vi "BRig_RT__Case_Exp__State_Selection.vi"(0 "input_state":T1, 2 "input_dataCurrent":u16[](array[numeric]), 3 "input_dataTrial":u16[][](array[numeric]), 4 "input_dataExp":u16[](array[numeric]), 5 "input_arrTrig":bool[](array[boolean]), 6 "input_FPGA_SelectWrong":bool, 8 "input_FPGA_SelectReward":bool, 10 "input_LickR":bool, 12 "input_LickL":bool) -> (7 "output_LC_Laser_l2":bool, 9 "output_LC_Event_l2":bool, 11 "output_LC_Laser_l1":bool, 13 "output_LC_Event_l1":bool, 14 "output_state":T1, 16 "output_dataCurrent":u16[](array[numeric]), 17 "output_dataTrial":u16[][](array[numeric]), 18 "output_anySelect_L":bool, 19 "output_anySelect_R":bool)   [LabVIEW 2014]
uses:
  myRIO_BRig_RT__Case_Exp_stateList.ctl
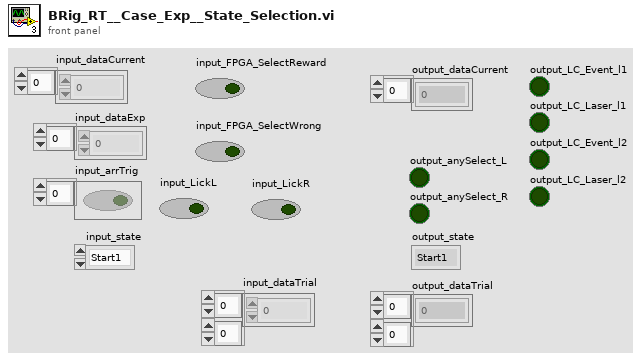
[diagram p1: front panel]
types:
  T1 = typedef "myRIO_BRig_RT__Case_Exp_stateList.ctl" = enum16{"Start1", "Start2", "Start3", "saveSettings1", "saveSettings2", "saveSettings3", "saveSettings4", "saveSettings_LC_ENL_l1", "saveSettings_LC_ENL_l2", "saveSettings_LC_Cue_l1", "saveSettings_LC_Cue_l2", "saveSettings6_LC_l1_Other", "SaveSettings6_LC_l2_Other", "setSettings_Audio", "setSettings_Laser", "initBlock_pre", "initBlock", "initBlock2", "initBlock_post", "initTrial_pre", "initTrial", "initTrial2", "initTrial3", "initTrial4", "initTrial_LC_ENL1", "initTrial_LC_Cue1", "initTrial_LC_Cue1_2", "initTrial_LC_Sel", "initTrial_post", "ENL1_pre", "ENL1", "ENL1_post", "ENL1Penalty_pre", "ENL1Penalty", "ENL2_pre", "ENL2", "ENL2Penalty_pre", "ENL2Penalty", "Cue1_pre", "Cue1", "Cue1_post", "Cue1Penalty_pre", "Cue1Penalty", "Cue2_pre", "Cue2", "Cue2Penalty_pre", "Cue2Penalty", "Selection_pre", "Selection", "Select_post", "SelectReward_pre", "SelectReward", "SelectRewardPost_pre", "SelectRewardPost", "SelectWrong_pre", "SelectWrong", "SelectWrong_post", "SelectTimeout_pre", "SelectTimeout", "SelectTimeout_post", "endTrial_pre", "endTrial1", "endTrial2", "endTrial3", "endTrial_post", "endBlock_pre", "endBlock", "endBlock_post", "endExp", "commConnect", "commUpload_pre", "commUpload_dataBlock", "commUpload_dataCurrent", "commUpload_dataExp", "commUpload_dataLC", "commUpload_dataTrial", "commUpload_post", "saveData_pre", "saveData_dataBlock", "saveData_dataCurrent", "saveData_dataExp", "saveData_dataLC", "saveData_dataTrial", "saveData_post", "empty_endBlock1", "empty_endBlock2", "empty_endTrial1", "empty_endTrial2", "empty_endTrial3", "empty_endTrial4", "empty_endTrial5", "dummyState", "dummyState_endBlock", "FreeReward_pre", "FreeReward", "FreeRewardPost_pre", "FreeRewardPost"}
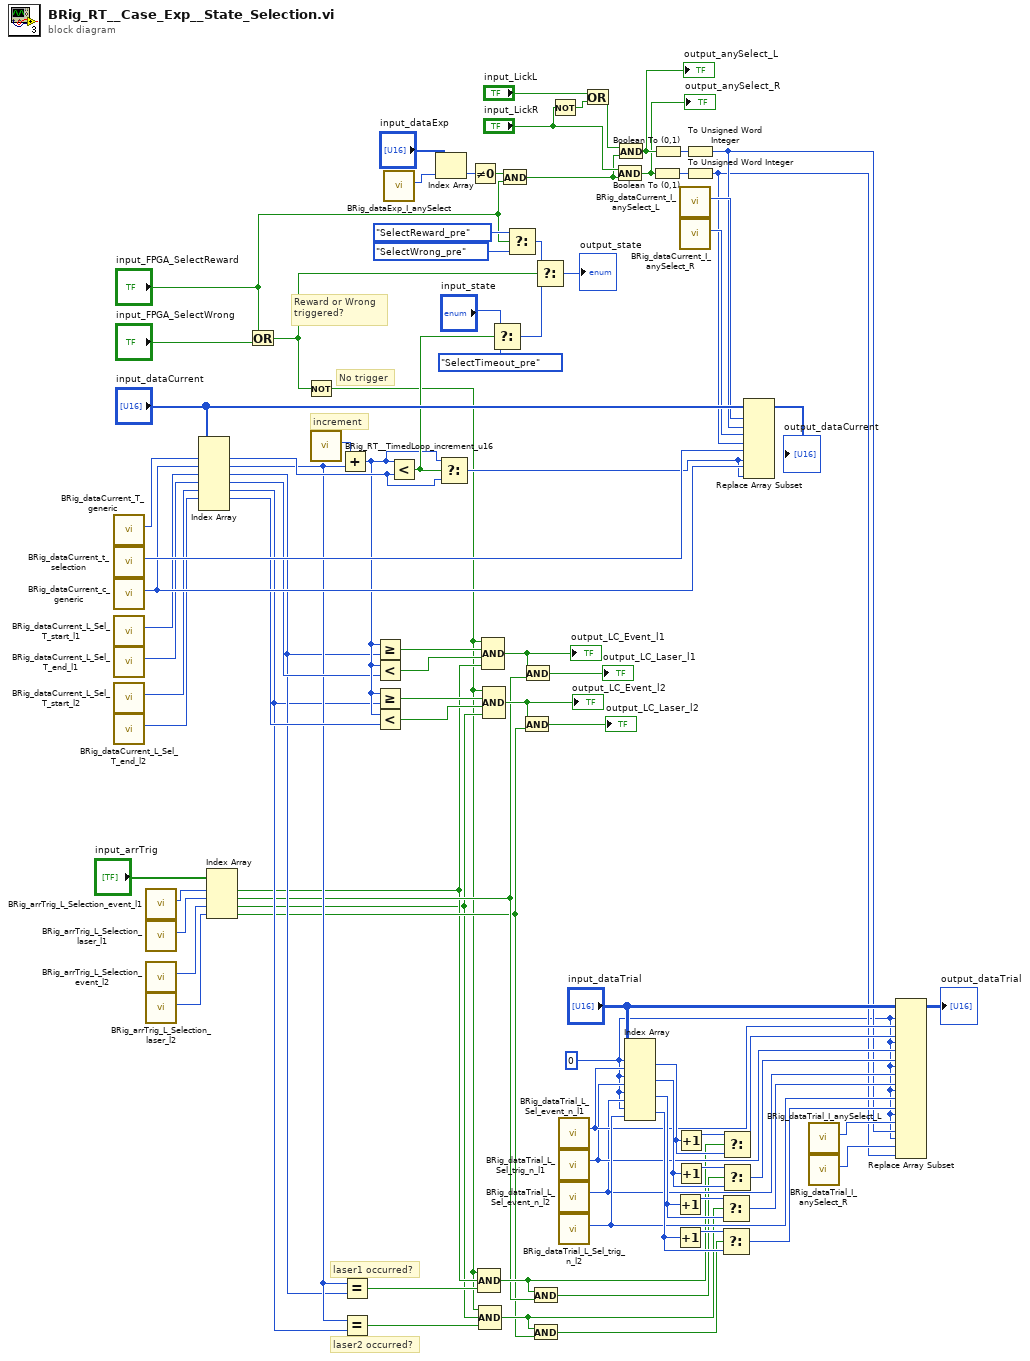
[diagram p0: block diagram]
diagram:
  w1 = 0
  # "No trigger"
  # "Reward or Wrong\ntriggered?"
  # "laser2 occurred?"
  # "laser1 occurred?"
  # "increment"
  n1 = call "BRig_dataCurrent_T_generic.vi"() -> ("output_T_generic"=w50:i32)  [unwired: 11 in]
  n2 = call "BRig_dataCurrent_t_selection.vi"() -> ("output_t_selection"=w49:i32)  [unwired: 11 in]
  n3 = call "BRig_dataCurrent_c_generic.vi"() -> ("output_count_generic"=w48:i32)  [unwired: 11 in]
  n4 = call "BRig_dataCurrent_L_Sel_T_start_l1.vi"() -> ("output_L_Sel_T_start_l1"=w45:i32)  [unwired: 11 in]
  n5 = call "BRig_dataCurrent_L_Sel_T_end_l1.vi"() -> ("output_L_Sel_T_end_l1"=w44:i32)  [unwired: 11 in]
  n6 = call "BRig_dataCurrent_L_Sel_T_start_l2.vi"() -> ("output_L_Sel_T_start_l2"=w43:i32)  [unwired: 11 in]
  n7 = call "BRig_dataCurrent_L_Sel_T_end_l2.vi"() -> ("output_L_Sel_T_end_l2"=w42:i32)  [unwired: 11 in]
  n8 = call "BRig_arrTrig_L_Selection_event_l1.vi"() -> ("output_L_Sel_event_l1"=w54:i32)  [unwired: 11 in]
  n9 = call "BRig_arrTrig_L_Selection_laser_l1.vi"() -> ("output_L_Sel_laserTrig_l1"=w55:i32)  [unwired: 11 in]
  n10 = call "BRig_arrTrig_L_Selection_event_l2.vi"() -> ("output_L_Sel_event_l2"=w56:i32)  [unwired: 11 in]
  n11 = call "BRig_arrTrig_L_Selection_laser_l2.vi"() -> ("output_L_Sel_laserTrig_l2"=w57:i32)  [unwired: 11 in]
  n12 = Index Array(array="input_dataCurrent", index #1=w50, index #2=w48, index #3=w45, index #4=w44, index #5=w43, index #6=w42) -> (element #1=w46:u16, element #2=w19:u16, element #3=w18:u16, element #4=w40:u16, element #5=w17:u16, element #6=w39:u16)  [unwired: 1 in, 1 out]
  n13 = Index Array(array="input_arrTrig", index #1=w54, index #2=w55, index #3=w56, index #4=w57) -> (element #1=w4:bool, element #2=w12:bool, element #3=w3:bool, element #4=w11:bool)
  n14 = Or(x="input_FPGA_SelectReward", y="input_FPGA_SelectWrong") -> (x .or. y?=w79:bool)
  n15 = Not(x=w79) -> (.not. x?=w2:bool)
  n16 = call "BRig_RT__TimedLoop_increment_u16.vi"() -> ("output_increment__u16"=w87:u16)  [unwired: 11 in]
  n17 = Add(x=w87, y=w19) -> (x+y=w41:u16)
  n18 = Equal?(x=w19, y=w18) -> (x = y?=w16:bool)
  n19 = Equal?(x=w19, y=w17) -> (x = y?=w15:bool)
  n20 = Greater Or Equal?(x=w41, y=w18) -> (x >= y?=w78:bool)
  n21 = Less?(x=w41, y=w40) -> (x < y?=w77:bool)
  n22 = Greater Or Equal?(x=w41, y=w17) -> (x >= y?=w75:bool)
  n23 = Less?(x=w41, y=w39) -> (x < y?=w74:bool)
  n24 = call "BRig_dataExp_I_anySelect.vi"() -> ("output_I_anySelect"=w67:i32)  [unwired: 11 in]
  n25 = Less?(x=w41, y=w46) -> (x < y?=w81:bool)
  n26 = Index Array(array="input_dataExp", index=w67) -> (element=w68:u16)
  n27 = Select(t=w41, s=w81, f=w46) -> (s? t:f=w47:u16)
  n28 = Not Equal To 0?(x=w68) -> (x != 0?=w53:bool)
  n29 = Compound Arithmetic op=AND(w2, w4, w16) -> (w14:bool)
  n30 = Compound Arithmetic op=AND(w2, w3, w15) -> (w13:bool)
  n31 = Compound Arithmetic op=AND(w2, w78, w77, w4) -> (w72:bool)
  "output_LC_Event_l1" <- w72
  n32 = Compound Arithmetic op=AND(w2, w75, w74, w3) -> (w73:bool)
  "output_LC_Event_l2" <- w73
  n33 = Select(t="input_state", s=w81, f=myRIO_BRig_RT__Case_Exp_stateList."SelectTimeout_pre" ("Enum")) -> (s? t:f=w84:T1)
  n34 = And(x=w53, y="input_FPGA_SelectReward") -> (x .and. y?=w51:bool)
  n35 = Select(t=myRIO_BRig_RT__Case_Exp_stateList."SelectReward_pre" ("Enum"), s="input_FPGA_SelectReward", f=myRIO_BRig_RT__Case_Exp_stateList."SelectWrong_pre" ("Enum")) -> (s? t:f=w88:T1)
  n36 = And(x=w73, y=w11) -> (x .and. y?=→"output_LC_Laser_l2":bool)
  n37 = And(x=w72, y=w12) -> (x .and. y?=→"output_LC_Laser_l1":bool)
  n38 = And(x=w14, y=w12) -> (x .and. y?=w10:bool)
  n39 = And(x=w13, y=w11) -> (x .and. y?=w9:bool)
  n40 = Select(t=w88, s=w79, f=w84) -> (s? t:f=→"output_state":T1)
  n41 = Not(x="input_LickR") -> (.not. x?=w59:bool)
  n42 = call "BRig_dataTrial_L_Sel_event_n_l1.vi"() -> ("output_L_Sel_event_n_l1"=w22:i32)  [unwired: 11 in]
  n43 = call "BRig_dataTrial_L_Sel_trig_n_l1.vi"() -> ("output_L_Sel_trig_n_l1"=w21:i32)  [unwired: 11 in]
  n44 = call "BRig_dataTrial_L_Sel_event_n_l2.vi"() -> ("output_L_Sel_event_n_l2"=w20:i32)  [unwired: 11 in]
  n45 = call "BRig_dataTrial_L_Sel_trig_n_l2.vi"() -> ("output_L_Sel_trig_n_l2"=w23:i32)  [unwired: 11 in]
  n46 = Or(x="input_LickL", y=w59) -> (x .or. y?=w58:bool)
  n47 = And(x="input_LickR", y=w51) -> (x .and. y?=w65:bool)
  "output_anySelect_R" <- w65
  n48 = And(x=w58, y=w51) -> (x .and. y?=w66:bool)
  "output_anySelect_L" <- w66
  n49 = Index Array(array="input_dataTrial", index (row) #1=w1, index (col) #1=w22, index (row) #2=w1, index (col) #2=w21, index (row) #3=w1, index (col) #3=w20, index (row) #4=w1, index (col) #4=w23) -> (element #1=w35:u16, element #2=w31:u16, element #3=w30:u16, element #4=w29:u16)
  n50 = Boolean To (0,1)(Boolean=w65) -> (0, 1=w63:i16)
  n51 = Boolean To (0,1)(Boolean=w66) -> (0, 1=w64:i16)
  n52 = Increment(x=w30) -> (x+1=w33:u16)
  n53 = Increment(x=w29) -> (x+1=w32:u16)
  n54 = Increment(x=w35) -> (x+1=w36:u16)
  n55 = Increment(x=w31) -> (x+1=w34:u16)
  n56 = call "BRig_dataCurrent_I_anySelect_L.vi"() -> ("output_IanySelect_L"=w62:i32)  [unwired: 11 in]
  n57 = call "BRig_dataCurrent_I_anySelect_R.vi"() -> ("output_IanySelect_R"=w61:i32)  [unwired: 11 in]
  n58 = To Unsigned Word Integer(number=w64) -> (unsigned 16bit integer=w6:u16)
  n59 = To Unsigned Word Integer(number=w63) -> (unsigned 16bit integer=w5:u16)
  n60 = Select(t=w33, s=w13, f=w30) -> (s? t:f=w26:u16)
  n61 = Select(t=w32, s=w9, f=w29) -> (s? t:f=w25:u16)
  n62 = Select(t=w36, s=w14, f=w35) -> (s? t:f=w28:u16)
  n63 = Select(t=w34, s=w10, f=w31) -> (s? t:f=w27:u16)
  n64 = Replace Array Subset(array="input_dataCurrent", new element #1=w6, index #1=w62, new element #2=w5, index #2=w61, new element #3=w47, index #3=w49, new element #4=w47, index #4=w48) -> (→"output_dataCurrent":u16[])
  n65 = call "BRig_dataTrial_I_anySelect_L.vi"() -> ("output_I_allReward_L"=w8:i32)  [unwired: 11 in]
  n66 = call "BRig_dataTrial_I_anySelect_R.vi"() -> ("output_I_anySelect_R"=w7:i32)  [unwired: 11 in]
  n67 = Replace Array Subset(array="input_dataTrial", new element #1=w28, index (row) #1=w1, index (col) #1=w22, new element #2=w27, index (row) #2=w1, index (col) #2=w21, new element #3=w26, index (row) #3=w1, index (col) #3=w20, new element #4=w25, index (row) #4=w1, index (col) #4=w23, new element #5=w6, index (row) #5=w1, index (col) #5=w8, new element #6=w5, index (row) #6=w1, index (col) #6=w7) -> (→"output_dataTrial":u16[][])
